vi "FindProjectItemsRecursive.vi"() -> ()   [LabVIEW 2013, in "ProjectHandler.lvlib"]
uses:
  ProjectHandler.lvlib
panel:
  out "error out":errorcluster
  in  "error in":errorcluster
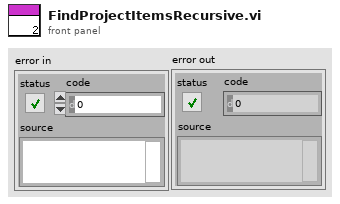
[diagram p1: front panel]
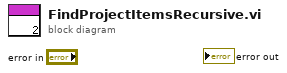
[diagram p0: block diagram]
diagram:
